vi "CAENHV Get Ch Param Bool.vi"(6 "ChList":u16[](array[numeric]), 7 "ChNum (1)":u16=1, 8 "error in (no error)":errorcluster, 9 "ParName":string, 10 "slot":u16, 11 "handle":i32) -> (0 "error out":errorcluster, 3 "ParValList":bool[](array[boolean]))   [LabVIEW 2018, in "CAENHVWrapper.lvlib"]
doc: "CAENHVLIB_API CAENHVRESULT CAENHV_GetChParam(int handle, ushort slot, \n const char *ParName, ushort ChNum, const ushort *ChList, void *ParValList);"
uses:
  CAENHVWrapper.lvlib
  CAEN SY5527  V2 NEW convention/data/CAENHVWrapper.dll
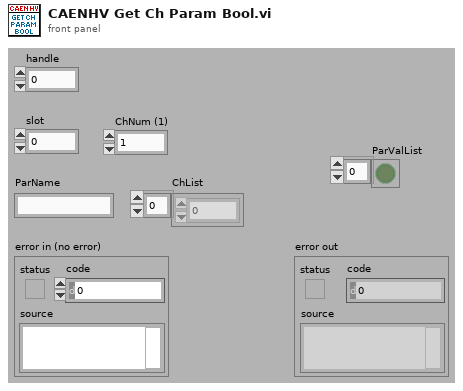
[diagram p1: front panel]
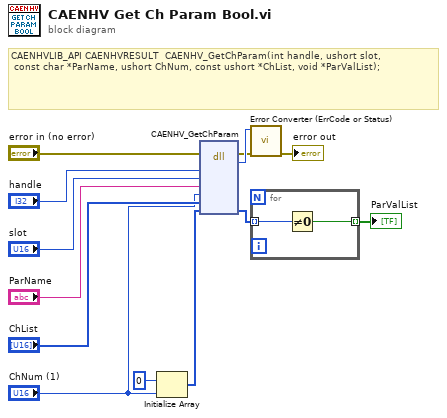
[diagram p0: block diagram]
diagram:
  # "CAENHVLIB_API CAENHVRESULT  CAENHV_GetChParam(int handle, ushort slot, \n const char *ParName, ushort ChNum, const ushort *ChList, void *ParValList);"
  n1 = Initialize Array(0 ("element"), "ChNum (1)") -> (w4:i32[])
  n2 = dll-call lib="C:/Users/Zaza/Desktop/SY5527 General soft 2018/CAEN SY5527  V2 NEW convention/data/CAENHVWrapper.*" fn="CAENHV_GetChParam"(error in="error in (no error)", "handle"="handle", "slot"="slot", "ParName"="ParName", "ChNum"="ChNum (1)", "ChList"="ChList", "ParValList"=w4) -> (error out=w8:errorcluster, "return type"=w9:i32, "ParValList"=w2:i32[])  [unwired: 7 in, 1 out]
  n3 = call "Error Converter (ErrCode or Status).vi"("error in (no error)"=w8, "error code"=w9) -> ("error out"=→"error out":errorcluster)  [unwired: 9 in]
  n4 = for {
    tunnel: w2 -> [w15] mode=indexing
    tunnel: [w14] -> w1 mode=indexing
    n5 = Not Equal To 0?(x=w15) -> (x != 0?=w14:bool)
  }
  "ParValList" <- w1
